vi "冰箱监测界面.vi"() -> ()   [LabVIEW 2016, in "环境动力监测库.lvlib"]
uses:
  <vilib>/ptbypt/NI_PtbyPt.lvlib
panel:
  out "关闭温度":dbl=40.0
  out "开启温度":dbl=50.0
  out "输出点":i32
  in  "控制开关":bool
  # "冰箱监测"
  # "℃"
  # "℃"
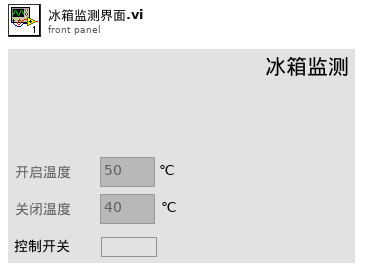
[diagram p1: front panel]
types:
  T1 = cluster{"环境变量":cluster{"蓄电池电压":dbl, "室温":dbl, "湿度":dbl, "水浸报警":bool, "烟雾报警":bool, "门禁1状态":bool, "门禁2状态":bool}, "ZLAN 6842 MB session":refnum<class "MB_Master.lvclass">, "DI":bool[], "DO":bool[]}
  T2 = cluster{"漏水监测配置":cluster{"监测项描述:输出":string, "端口":enum16{"AI0", "AI1", "AI2", "AI3", "AI4", "DI0", "DI1", "DI2", "DI3", "DI4", "DI5", "DI6", "DI7", "DO0", "DO1", "DO2", "DO3", "DO4", "DO5", "DO6", "DO7", "X0", "X1", "X2", "X3", "X4", "X5", "X6", "X7", "X8", "X9", "X10", "X11", "X12", "X13", "X14", "X15", "X16", "X17", "X18", "X19", "X20", "X21", "X22", "X23", "Y0", "Y1", "Y2", "Y3", "Y4", "Y5", "Y6", "Y7", "Y8", "Y9", "Y10", "Y11", "Y12", "Y13", "Y14", "Y15", "Y16", "Y17", "Y18", "Y19", "Y20", "Y21", "Y22", "Y23", "Y24", "Y25", "Y26", "Y27", "Y28", "Y29", "Y30", "Y31", "Y32", "Y33", "Y34", "Y35", "Y36", "Y37", "Y38", "Y39"}, "告警参数:":enum32{"禁用告警", "闭合告警", "断开告警"}, "传感器型号:":enum16{"PLC", "ZLAN", "ART"}, "声光告警启用":bool}, "门禁开关监测配置":cluster{"监测项描述:输出":string, "端口":enum16{"AI0", "AI1", "AI2", "AI3", "AI4", "DI0", "DI1", "DI2", "DI3", "DI4", "DI5", "DI6", "DI7", "DO0", "DO1", "DO2", "DO3", "DO4", "DO5", "DO6", "DO7", "X0", "X1", "X2", "X3", "X4", "X5", "X6", "X7", "X8", "X9", "X10", "X11", "X12", "X13", "X14", "X15", "X16", "X17", "X18", "X19", "X20", "X21", "X22", "X23", "Y0", "Y1", "Y2", "Y3", "Y4", "Y5", "Y6", "Y7", "Y8", "Y9", "Y10", "Y11", "Y12", "Y13", "Y14", "Y15", "Y16", "Y17", "Y18", "Y19", "Y20", "Y21", "Y22", "Y23", "Y24", "Y25", "Y26", "Y27", "Y28", "Y29", "Y30", "Y31", "Y32", "Y33", "Y34", "Y35", "Y36", "Y37", "Y38", "Y39"}, "告警参数:":enum32{"禁用告警", "闭合告警", "断开告警"}, "传感器型号:":enum16{"PLC", "ZLAN", "ART"}, "声光告警启用":bool}, "门禁开关监测配置2":cluster{"监测项描述:输出":string, "端口":enum16{"AI0", "AI1", "AI2", "AI3", "AI4", "DI0", "DI1", "DI2", "DI3", "DI4", "DI5", "DI6", "DI7", "DO0", "DO1", "DO2", "DO3", "DO4", "DO5", "DO6", "DO7", "X0", "X1", "X2", "X3", "X4", "X5", "X6", "X7", "X8", "X9", "X10", "X11", "X12", "X13", "X14", "X15", "X16", "X17", "X18", "X19", "X20", "X21", "X22", "X23", "Y0", "Y1", "Y2", "Y3", "Y4", "Y5", "Y6", "Y7", "Y8", "Y9", "Y10", "Y11", "Y12", "Y13", "Y14", "Y15", "Y16", "Y17", "Y18", "Y19", "Y20", "Y21", "Y22", "Y23", "Y24", "Y25", "Y26", "Y27", "Y28", "Y29", "Y30", "Y31", "Y32", "Y33", "Y34", "Y35", "Y36", "Y37", "Y38", "Y39"}, "告警参数:":enum32{"禁用告警", "闭合告警", "断开告警"}, "传感器型号:":enum16{"PLC", "ZLAN", "ART"}, "声光告警启用":bool}, "温湿度监测配置":cluster{"监测项描述:输出":string, "端口":enum16{"AI0", "AI1", "AI2", "AI3", "AI4", "DI0", "DI1", "DI2", "DI3", "DI4", "DI5", "DI6", "DI7", "DO0", "DO1", "DO2", "DO3", "DO4", "DO5", "DO6", "DO7", "X0", "X1", "X2", "X3", "X4", "X5", "X6", "X7", "X8", "X9", "X10", "X11", "X12", "X13", "X14", "X15", "X16", "X17", "X18", "X19", "X20", "X21", "X22", "X23", "Y0", "Y1", "Y2", "Y3", "Y4", "Y5", "Y6", "Y7", "Y8", "Y9", "Y10", "Y11", "Y12", "Y13", "Y14", "Y15", "Y16", "Y17", "Y18", "Y19", "Y20", "Y21", "Y22", "Y23", "Y24", "Y25", "Y26", "Y27", "Y28", "Y29", "Y30", "Y31", "Y32", "Y33", "Y34", "Y35", "Y36", "Y37", "Y38", "Y39"}, "告警参数:":enum32{"禁用告警", "闭合告警", "断开告警"}, "传感器型号:":enum16{"PLC", "ZLAN", "ART"}, "声光告警启用":bool}, "烟雾监测配置":cluster{"监测项描述:输出":string, "端口":enum16{"AI0", "AI1", "AI2", "AI3", "AI4", "DI0", "DI1", "DI2", "DI3", "DI4", "DI5", "DI6", "DI7", "DO0", "DO1", "DO2", "DO3", "DO4", "DO5", "DO6", "DO7", "X0", "X1", "X2", "X3", "X4", "X5", "X6", "X7", "X8", "X9", "X10", "X11", "X12", "X13", "X14", "X15", "X16", "X17", "X18", "X19", "X20", "X21", "X22", "X23", "Y0", "Y1", "Y2", "Y3", "Y4", "Y5", "Y6", "Y7", "Y8", "Y9", "Y10", "Y11", "Y12", "Y13", "Y14", "Y15", "Y16", "Y17", "Y18", "Y19", "Y20", "Y21", "Y22", "Y23", "Y24", "Y25", "Y26", "Y27", "Y28", "Y29", "Y30", "Y31", "Y32", "Y33", "Y34", "Y35", "Y36", "Y37", "Y38", "Y39"}, "告警参数:":enum32{"禁用告警", "闭合告警", "断开告警"}, "传感器型号:":enum16{"PLC", "ZLAN", "ART"}, "声光告警启用":bool}, "冰箱监测配置":cluster{"监测项描述:输出":string, "端口":enum16{"AI0", "AI1", "AI2", "AI3", "AI4", "DI0", "DI1", "DI2", "DI3", "DI4", "DI5", "DI6", "DI7", "DO0", "DO1", "DO2", "DO3", "DO4", "DO5", "DO6", "DO7", "X0", "X1", "X2", "X3", "X4", "X5", "X6", "X7", "X8", "X9", "X10", "X11", "X12", "X13", "X14", "X15", "X16", "X17", "X18", "X19", "X20", "X21", "X22", "X23", "Y0", "Y1", "Y2", "Y3", "Y4", "Y5", "Y6", "Y7", "Y8", "Y9", "Y10", "Y11", "Y12", "Y13", "Y14", "Y15", "Y16", "Y17", "Y18", "Y19", "Y20", "Y21", "Y22", "Y23", "Y24", "Y25", "Y26", "Y27", "Y28", "Y29", "Y30", "Y31", "Y32", "Y33", "Y34", "Y35", "Y36", "Y37", "Y38", "Y39"}, "告警参数:":enum32{"禁用告警", "闭合告警", "断开告警"}, "传感器型号:":enum16{"PLC", "ZLAN", "ART"}, "声光告警启用":bool}, "排气扇监测配置":cluster{"监测项描述:输出":string, "端口":enum16{"AI0", "AI1", "AI2", "AI3", "AI4", "DI0", "DI1", "DI2", "DI3", "DI4", "DI5", "DI6", "DI7", "DO0", "DO1", "DO2", "DO3", "DO4", "DO5", "DO6", "DO7", "X0", "X1", "X2", "X3", "X4", "X5", "X6", "X7", "X8", "X9", "X10", "X11", "X12", "X13", "X14", "X15", "X16", "X17", "X18", "X19", "X20", "X21", "X22", "X23", "Y0", "Y1", "Y2", "Y3", "Y4", "Y5", "Y6", "Y7", "Y8", "Y9", "Y10", "Y11", "Y12", "Y13", "Y14", "Y15", "Y16", "Y17", "Y18", "Y19", "Y20", "Y21", "Y22", "Y23", "Y24", "Y25", "Y26", "Y27", "Y28", "Y29", "Y30", "Y31", "Y32", "Y33", "Y34", "Y35", "Y36", "Y37", "Y38", "Y39"}, "告警参数:":enum32{"禁用告警", "闭合告警", "断开告警"}, "传感器型号:":enum16{"PLC", "ZLAN", "ART"}, "声光告警启用":bool}, "红外入侵监测配置":cluster{"监测项描述:输出":string, "端口":enum16{"AI0", "AI1", "AI2", "AI3", "AI4", "DI0", "DI1", "DI2", "DI3", "DI4", "DI5", "DI6", "DI7", "DO0", "DO1", "DO2", "DO3", "DO4", "DO5", "DO6", "DO7", "X0", "X1", "X2", "X3", "X4", "X5", "X6", "X7", "X8", "X9", "X10", "X11", "X12", "X13", "X14", "X15", "X16", "X17", "X18", "X19", "X20", "X21", "X22", "X23", "Y0", "Y1", "Y2", "Y3", "Y4", "Y5", "Y6", "Y7", "Y8", "Y9", "Y10", "Y11", "Y12", "Y13", "Y14", "Y15", "Y16", "Y17", "Y18", "Y19", "Y20", "Y21", "Y22", "Y23", "Y24", "Y25", "Y26", "Y27", "Y28", "Y29", "Y30", "Y31", "Y32", "Y33", "Y34", "Y35", "Y36", "Y37", "Y38", "Y39"}, "告警参数:":enum32{"禁用告警", "闭合告警", "断开告警"}, "传感器型号:":enum16{"PLC", "ZLAN", "ART"}, "声光告警启用":bool}, "振动监测配置":cluster{"监测项描述:输出":string, "端口":enum16{"AI0", "AI1", "AI2", "AI3", "AI4", "DI0", "DI1", "DI2", "DI3", "DI4", "DI5", "DI6", "DI7", "DO0", "DO1", "DO2", "DO3", "DO4", "DO5", "DO6", "DO7", "X0", "X1", "X2", "X3", "X4", "X5", "X6", "X7", "X8", "X9", "X10", "X11", "X12", "X13", "X14", "X15", "X16", "X17", "X18", "X19", "X20", "X21", "X22", "X23", "Y0", "Y1", "Y2", "Y3", "Y4", "Y5", "Y6", "Y7", "Y8", "Y9", "Y10", "Y11", "Y12", "Y13", "Y14", "Y15", "Y16", "Y17", "Y18", "Y19", "Y20", "Y21", "Y22", "Y23", "Y24", "Y25", "Y26", "Y27", "Y28", "Y29", "Y30", "Y31", "Y32", "Y33", "Y34", "Y35", "Y36", "Y37", "Y38", "Y39"}, "告警参数:":enum32{"禁用告警", "闭合告警", "断开告警"}, "传感器型号:":enum16{"PLC", "ZLAN", "ART"}, "声光告警启用":bool}, "废液监测配置":cluster{"监测项描述:输出":string, "端口":enum16{"AI0", "AI1", "AI2", "AI3", "AI4", "DI0", "DI1", "DI2", "DI3", "DI4", "DI5", "DI6", "DI7", "DO0", "DO1", "DO2", "DO3", "DO4", "DO5", "DO6", "DO7", "X0", "X1", "X2", "X3", "X4", "X5", "X6", "X7", "X8", "X9", "X10", "X11", "X12", "X13", "X14", "X15", "X16", "X17", "X18", "X19", "X20", "X21", "X22", "X23", "Y0", "Y1", "Y2", "Y3", "Y4", "Y5", "Y6", "Y7", "Y8", "Y9", "Y10", "Y11", "Y12", "Y13", "Y14", "Y15", "Y16", "Y17", "Y18", "Y19", "Y20", "Y21", "Y22", "Y23", "Y24", "Y25", "Y26", "Y27", "Y28", "Y29", "Y30", "Y31", "Y32", "Y33", "Y34", "Y35", "Y36", "Y37", "Y38", "Y39"}, "告警参数:":enum32{"禁用告警", "闭合告警", "断开告警"}, "传感器型号:":enum16{"PLC", "ZLAN", "ART"}, "声光告警启用":bool}, "废液监测配置2":cluster{"监测项描述:输出":string, "端口":enum16{"AI0", "AI1", "AI2", "AI3", "AI4", "DI0", "DI1", "DI2", "DI3", "DI4", "DI5", "DI6", "DI7", "DO0", "DO1", "DO2", "DO3", "DO4", "DO5", "DO6", "DO7", "X0", "X1", "X2", "X3", "X4", "X5", "X6", "X7", "X8", "X9", "X10", "X11", "X12", "X13", "X14", "X15", "X16", "X17", "X18", "X19", "X20", "X21", "X22", "X23", "Y0", "Y1", "Y2", "Y3", "Y4", "Y5", "Y6", "Y7", "Y8", "Y9", "Y10", "Y11", "Y12", "Y13", "Y14", "Y15", "Y16", "Y17", "Y18", "Y19", "Y20", "Y21", "Y22", "Y23", "Y24", "Y25", "Y26", "Y27", "Y28", "Y29", "Y30", "Y31", "Y32", "Y33", "Y34", "Y35", "Y36", "Y37", "Y38", "Y39"}, "告警参数:":enum32{"禁用告警", "闭合告警", "断开告警"}, "传感器型号:":enum16{"PLC", "ZLAN", "ART"}, "声光告警启用":bool}}
  T3 = cluster{"监测项描述:输出":string, "端口":enum16{"AI0", "AI1", "AI2", "AI3", "AI4", "DI0", "DI1", "DI2", "DI3", "DI4", "DI5", "DI6", "DI7", "DO0", "DO1", "DO2", "DO3", "DO4", "DO5", "DO6", "DO7", "X0", "X1", "X2", "X3", "X4", "X5", "X6", "X7", "X8", "X9", "X10", "X11", "X12", "X13", "X14", "X15", "X16", "X17", "X18", "X19", "X20", "X21", "X22", "X23", "Y0", "Y1", "Y2", "Y3", "Y4", "Y5", "Y6", "Y7", "Y8", "Y9", "Y10", "Y11", "Y12", "Y13", "Y14", "Y15", "Y16", "Y17", "Y18", "Y19", "Y20", "Y21", "Y22", "Y23", "Y24", "Y25", "Y26", "Y27", "Y28", "Y29", "Y30", "Y31", "Y32", "Y33", "Y34", "Y35", "Y36", "Y37", "Y38", "Y39"}, "告警参数:":enum32{"禁用告警", "闭合告警", "断开告警"}, "传感器型号:":enum16{"PLC", "ZLAN", "ART"}, "声光告警启用":bool}
  T4 = enum16{"AI0", "AI1", "AI2", "AI3", "AI4", "DI0", "DI1", "DI2", "DI3", "DI4", "DI5", "DI6", "DI7", "DO0", "DO1", "DO2", "DO3", "DO4", "DO5", "DO6", "DO7", "X0", "X1", "X2", "X3", "X4", "X5", "X6", "X7", "X8", "X9", "X10", "X11", "X12", "X13", "X14", "X15", "X16", "X17", "X18", "X19", "X20", "X21", "X22", "X23", "Y0", "Y1", "Y2", "Y3", "Y4", "Y5", "Y6", "Y7", "Y8", "Y9", "Y10", "Y11", "Y12", "Y13", "Y14", "Y15", "Y16", "Y17", "Y18", "Y19", "Y20", "Y21", "Y22", "Y23", "Y24", "Y25", "Y26", "Y27", "Y28", "Y29", "Y30", "Y31", "Y32", "Y33", "Y34", "Y35", "Y36", "Y37", "Y38", "Y39"}
  T5 = cluster{"温湿度":cluster{"状态":bool, "温度:":sgl, "湿度:":sgl, "详情  ":bool}, "空调":cluster{"状态":bool, "机柜温度:":sgl, "压缩机:":enum16{"停止", "运行"}, "电加热:":enum16{"停止", "运行"}, "详情  ":bool}, "排气扇":cluster{"排气扇":bool, "详情  ":bool}, "冰箱":cluster{"冰箱":bool, "详情  ":bool}}
  T6 = cluster{"状态":cluster{"R0":i16, "R1":i16, "R2":i16, "R3":i16, "R4":i16, "R5":i16, "R6":i16, "R7":i16, "R8":i16, "R9":i16, "R10":i16, "R11":i16, "R12":i16, "R13":i16, "R14":i16, "R15":i16, "R16":i16, "R17":i16, "R18":i16, "R19":i16, "R20":i16, "R21":i16, "R22":i16, "R23":i16, "R24":i16, "R25":i16, "R26":i16, "R27":i16, "R28":i16, "R29":i16, "R30":i16, "R31":i16, "R32":i16, "R33":i16, "R34":i16, "R35":i16, "R36":i16, "R37":i16, "R38":i16, "R39":i16}, "输入状态":bool[], "输出状态":bool[], "参数设置":cluster{"R100":i16, "R101":i16, "R102":i16, "R103":i16, "R104":i16, "R105":i16, "R106":i16, "R107":i16, "R108":i16, "R109":i16, "R110":i16, "R111":i16, "R112":i16, "R113":i16, "R114":i16, "R115":i16, "R116":i16, "R117":i16, "R118":i16, "R119":i16, "R120":i16, "R121":i16, "R122":i16, "R123":i16}, "转换值":cluster{"AD0":sgl, "AD1":sgl, "AD2":sgl, "AD3":sgl, "AD4":sgl, "AD5":sgl}}
  T7 = cluster{"状态":cluster{"R0":i16, "R1":i16, "R2":i16, "R3":i16, "R4":i16, "R5":i16, "R6":i16, "R7":i16, "R8":i16, "R9":i16, "R10":i16, "R11":i16, "R12":i16, "R13":i16, "R14":i16, "R15":i16, "R16":i16, "R17":i16, "R18":i16, "R19":i16, "R20":i16, "R21":i16, "R22":i16, "R23":i16, "R24":i16, "R25":i16, "R26":i16, "R27":i16, "R28":i16, "R29":i16, "R30":i16, "R31":i16, "R32":i16, "R33":i16, "R34":i16, "R35":i16, "R36":i16, "R37":i16, "R38":i16, "R39":i16, "R40":i16, "R41":i16, "R42":i16, "R43":i16, "R44":i16, "R45":i16, "R46":i16, "R47":i16, "R48":i16, "R49":i16, "R50":i16, "R51":i16, "R52":i16, "R53":i16, "R54":i16, "R55":i16, "R56":i16, "R57":i16, "R58":i16, "R59":i16, "R60":i16, "R61":i16, "R62":i16, "R63":i16, "R64":i16, "R65":i16, "R66":i16, "R67":i16, "R68":i16, "R69":i16}, "输入状态":bool[], "输出状态":bool[], "报警簇":bool[], "参数设置":cluster{"R100":i16, "R101":i16, "R102":i16, "R103":i16, "R104":i16, "R105":i16, "R106":i16, "R107":i16, "R108":i16, "R109":i16, "R110":i16, "R111":i16, "R112":i16, "R113":i16, "R114":i16, "R115":i16, "R116":i16, "R117":i16, "R118":i16, "R119":i16, "R120":i16, "R121":i16, "R122":i16, "R123":i16, "R124":i16}, "转换值":cluster{"AD0":sgl, "AD1":sgl, "AD2":sgl, "AD3":sgl, "AD4":sgl, "AD5":sgl}, "看门狗启用":bool, "氨氮模块名称":string, "总磷模块名称":string, "采配水模块类型":enum16{"V1", "V2", "V3", "V4", "室内V1", "室内V2"}}
  T8 = cluster{"AD0":dbl, "AD1":dbl, "AD2":dbl, "AD3":dbl, "AD4":dbl, "AD5":dbl, "AD6":dbl, "AD7":dbl}
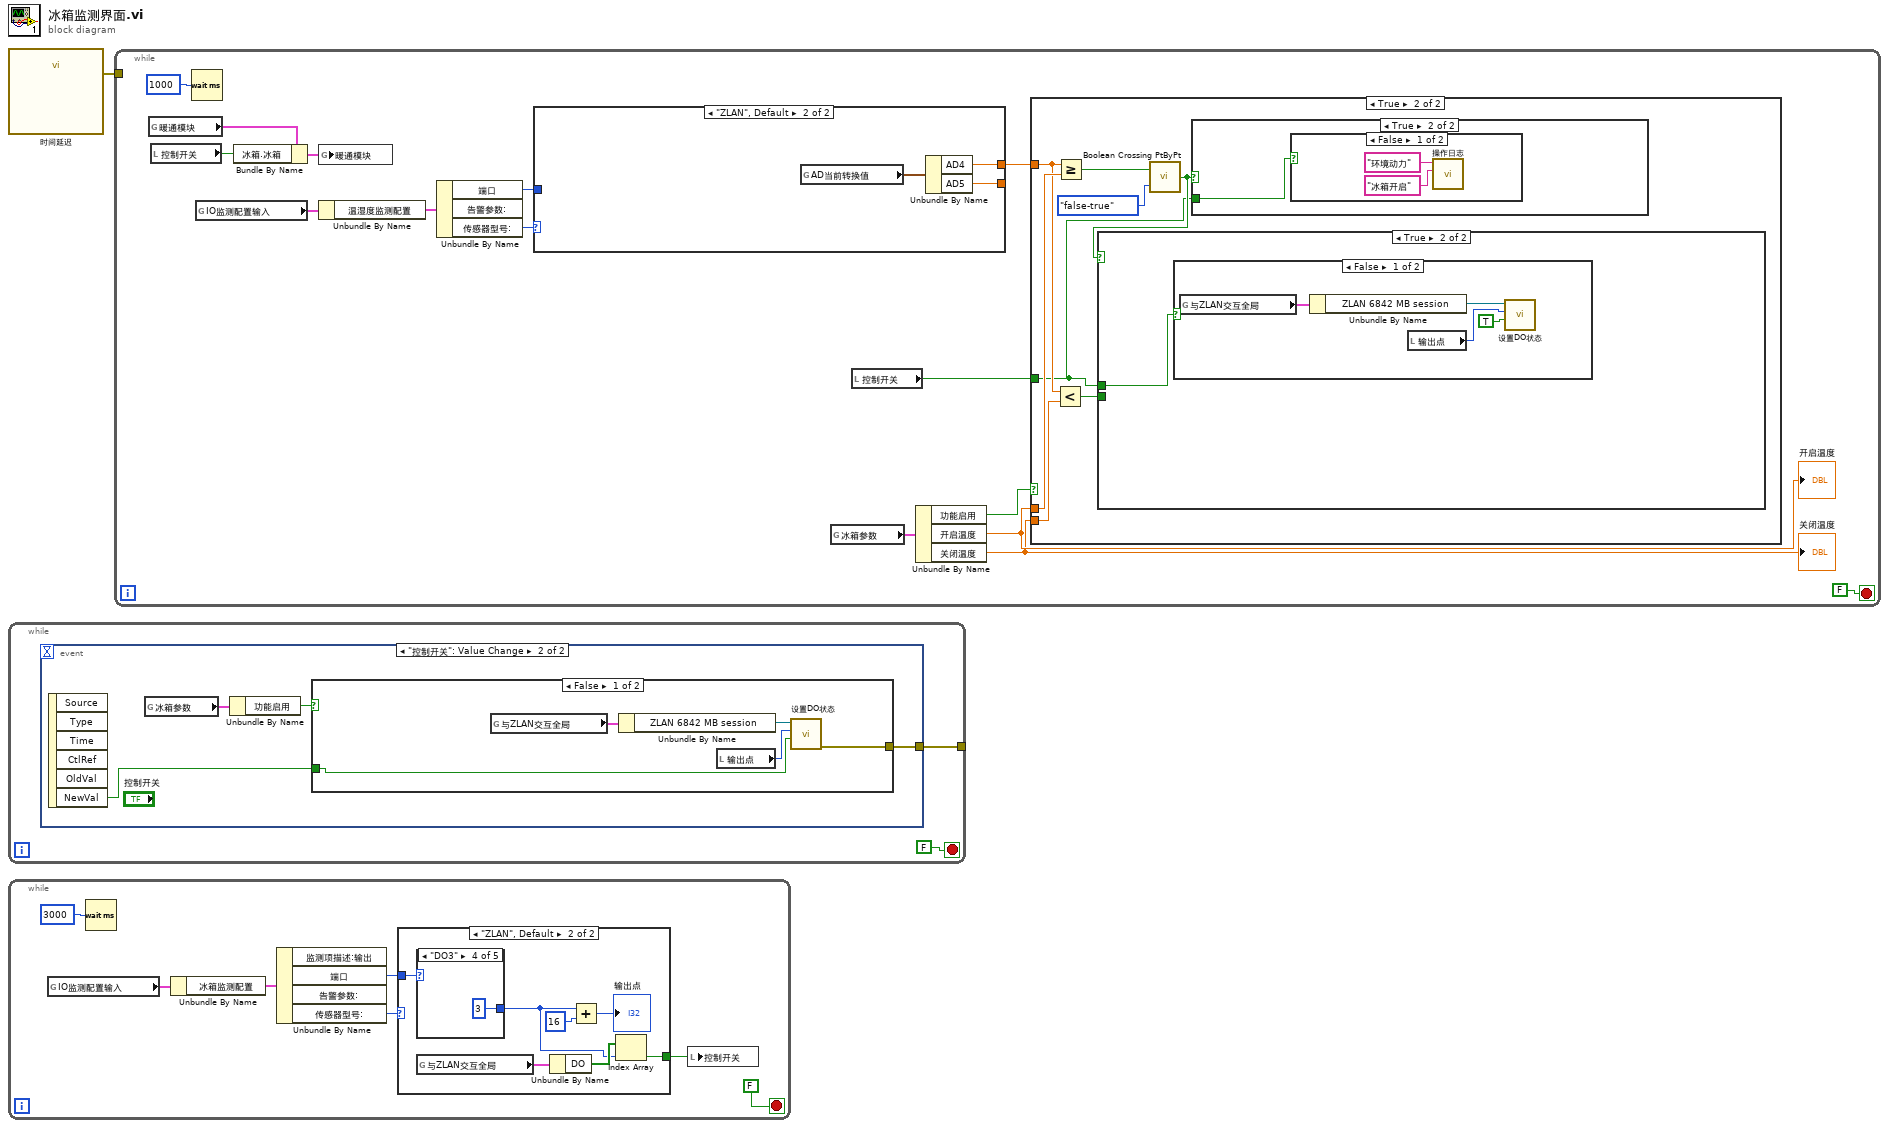
[diagram p0: block diagram]
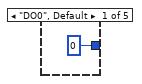
[diagram p3: hidden frame]
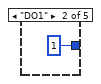
[diagram p4: hidden frame]
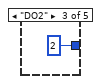
[diagram p5: hidden frame]
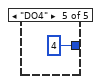
[diagram p6: hidden frame]
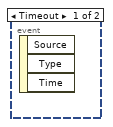
[diagram p7: hidden frame]
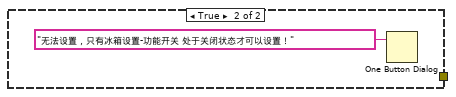
[diagram p8: hidden frame]
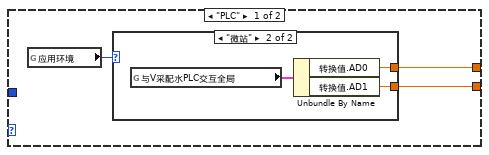
[diagram p9: hidden frame]
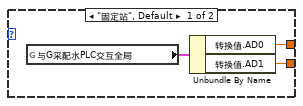
[diagram p10: hidden frame]
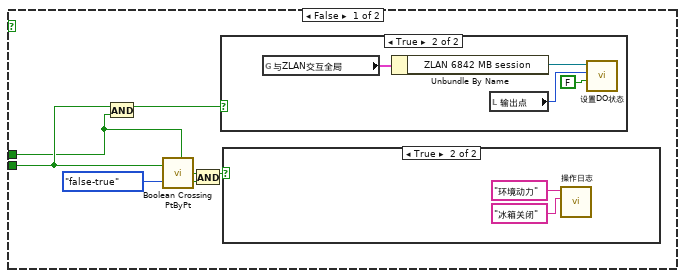
[diagram p12: hidden frame]
diagram:
  n1 = call "时间延迟"() -> ("error out"=w1:errorcluster)  [unwired: 11 in]
  n2 = while {
    tunnel: [w2] -> _
    stop <- FALSE stop-if-true
    n3 = event shown="[1] \"控制开关\": Value Change" {
      selector: _ -> [_ _]
      dyn-events: _ -> [_ _]
      timeout: _ -> [_ _]
      tunnel: [_ w4] -> w2
      event Timeout {
        n4 = event-data() -> ()  [unwired: 1 in, 3 out]
      }
      event "控制开关": Value Change {
        n5 = event-data() -> ("NewVal"=w5:bool)  [unwired: 1 in, 5 out]
        n6 = global read "断电保存全局变量.vi" "冰箱参数"() -> (w7:cluster{"功能启用":bool, "开启温度":dbl, "关闭温度":dbl})
        n7 = Unbundle By Name(w7) -> ("功能启用"=w6:bool)
        n8 = case shown="False" w6 {
          tunnel: w5 -> [w12 _]
          tunnel: [w11 _] -> w4
          frame False {
            n9 = global read "外部交互全局变量.vi" "与ZLAN交互全局"() -> (w10:T1)
            n10 = Unbundle By Name(w10) -> ("ZLAN 6842 MB session"=w9:refnum<class "MB_Master.lvclass">)
            n11 = local read "输出点"() -> (w8:i32)
            n12 = call "设置DO状态.vi"("value"=w12, "address"=w8, "MB session in"=w9) -> ("error out"=w11:errorcluster)  [unwired: 7 in, 1 out]
          }
          frame True {
            n13 = One Button Dialog(message="无法设置，只有冰箱设置-功能开关 处于关闭状态才可以设置！" ("消息")) -> ()  [unwired: 1 in, 1 out]
          }
        }
      }
    }
  }
  n14 = while {
    stop <- FALSE stop-if-true
    n15 = global read "断电保存全局变量.vi" "IO监测配置输入"() -> (w18:T2)
    n16 = Wait (ms)(milliseconds to wait=u32 3000 ("等待时间（毫秒）")) -> ()  [unwired: 1 out]
    n17 = Unbundle By Name(w18) -> ("冰箱监测配置"=w14:T3)
    n18 = Unbundle By Name(w14) -> ("端口"=w15:T4, "传感器型号:"=w16:enum16{"PLC", "ZLAN", "ART"})  [unwired: 2 out]
    n19 = case shown="\"ZLAN\", Default" w16 {
      tunnel: w15 -> [_ w27]
      tunnel: [_ w26] -> w17
      frame "PLC" {
      }
      frame "ZLAN", Default {
        n20 = case shown="\"DO3\"" w27 {
          tunnel: [0 1 2 3 4] -> w21
          frame "DO0", Default {
          }
          frame "DO1" {
          }
          frame "DO2" {
          }
          frame "DO3" {
          }
          frame "DO4" {
          }
        }
        n21 = global read "外部交互全局变量.vi" "与ZLAN交互全局"() -> (w25:T1)
        n22 = Unbundle By Name(w25) -> ("DO"=w24:bool[])
        n23 = Add(x=w21, y=16) -> (x+y=→"输出点":i32)
        n24 = Index Array(array=w24, index=w21) -> (element=w26:bool)
      }
    }
    n25 = local write "控制开关"(w17) -> ()
  }
  n26 = while {
    tunnel: w1 -> [_]
    stop <- FALSE stop-if-true
    n27 = global read "内部交互全局变量.vi" "暖通模块"() -> (w43:T5)
    n28 = local read "控制开关"() -> (w41:bool)
    n29 = Wait (ms)(milliseconds to wait=u32 1000 ("等待时间（毫秒）")) -> ()  [unwired: 1 out]
    n30 = global read "断电保存全局变量.vi" "IO监测配置输入"() -> (w36:T2)
    n31 = Bundle By Name(cluster=w43, "冰箱.冰箱"=w41) -> (w42:T5)
    n32 = global write "内部交互全局变量.vi" "暖通模块"(w42) -> ()
    n33 = Unbundle By Name(w36) -> ("温湿度监测配置"=w38:T3)
    n34 = Unbundle By Name(w38) -> ("端口"=w35:T4, "传感器型号:"=w37:enum16{"PLC", "ZLAN", "ART"})  [unwired: 1 out]
    n35 = case shown="\"ZLAN\", Default" w37 {
      tunnel: w35 -> [_ _]
      tunnel: [w49 w58] -> w34
      tunnel: [w48 w57] -> _
      frame "PLC" {
        n36 = global read "外部交互全局变量.vi" "应用环境"() -> (w50:enum16{"固定站", "微站", "浮标", "浮船"})
        n37 = case shown="\"微站\"" w50 {
          tunnel: [w52 w55] -> w49
          tunnel: [w51 w54] -> w48
          frame "固定站", Default {
            n38 = global read "外部交互全局变量.vi" "与G采配水PLC交互全局"() -> (w53:T6)
            n39 = Unbundle By Name(w53) -> ("转换值.AD0"=w52:sgl, "转换值.AD1"=w51:sgl)
          }
          frame "微站" {
            n40 = global read "外部交互全局变量.vi" "与V采配水PLC交互全局"() -> (w56:T7)
            n41 = Unbundle By Name(w56) -> ("转换值.AD0"=w55:sgl, "转换值.AD1"=w54:sgl)
          }
        }
      }
      frame "ZLAN", Default {
        n42 = global read "断电保存全局变量.vi" "AD当前转换值"() -> (w59:T8)
        n43 = Unbundle By Name(w59) -> ("AD4"=w58:dbl, "AD5"=w57:dbl)
      }
    }
    n44 = global read "断电保存全局变量.vi" "冰箱参数"() -> (w45:cluster{"功能启用":bool, "开启温度":dbl, "关闭温度":dbl})
    n45 = local read "控制开关"() -> (w33:bool)
    n46 = Unbundle By Name(w45) -> ("功能启用"=w44:bool, "开启温度"=w40:dbl, "关闭温度"=w39:dbl)
    "开启温度" <- w40
    "关闭温度" <- w39
    n47 = case shown="True" w44 {
      tunnel: w40 -> [_ w66]
      tunnel: w39 -> [_ w63]
      tunnel: w34 -> [_ w64]
      tunnel: w33 -> [_ w60]
      frame False {
      }
      frame True {
        n48 = Less?(x=w64, y=w63) -> (x < y?=w62:bool)
        n49 = Greater Or Equal?(x=w64, y=w66) -> (x >= y?=w65:bool)
        n50 = call <vilib>:"Boolean Crossing PtByPt.vi"("direction"=enum16{"either", "false-true", "true-false"}."false-true", "input"=w65) -> ("crossing"=w61:bool)  [unwired: 1 in]
        n51 = case shown="True" w61 {
          tunnel: w62 -> [w71 _]
          tunnel: w60 -> [w68 w80]
          frame False {
            n52 = And(x=w71, y=w68) -> (x .and. y?=w70:bool)
            n53 = call <vilib>:"Boolean Crossing PtByPt.vi"("direction"=enum16{"either", "false-true", "true-false"}."false-true", "input"=w71) -> ("crossing"=w72:bool)  [unwired: 1 in]
            n54 = And(x=w72, y=w68) -> (x .and. y?=w69:bool)
            n55 = case shown="True" w70 {
              frame False {
              }
              frame True {
                n56 = global read "外部交互全局变量.vi" "与ZLAN交互全局"() -> (w75:T1)
                n57 = Unbundle By Name(w75) -> ("ZLAN 6842 MB session"=w76:refnum<class "MB_Master.lvclass">)
                n58 = local read "输出点"() -> (w77:i32)
                n59 = call "设置DO状态.vi"("value"=FALSE, "address"=w77, "MB session in"=w76) -> ()  [unwired: 7 in, 2 out]
              }
            }
            n60 = case shown="True" w69 {
              frame False {
              }
              frame True {
                n61 = call "操作日志.vi"("日志信息"="冰箱关闭" ("设备"), "设备"="环境动力") -> ()  [unwired: 9 in, 1 out]
              }
            }
          }
          frame True {
            n62 = case shown="False" w80 {
              frame False {
                n63 = global read "外部交互全局变量.vi" "与ZLAN交互全局"() -> (w82:T1)
                n64 = Unbundle By Name(w82) -> ("ZLAN 6842 MB session"=w83:refnum<class "MB_Master.lvclass">)
                n65 = local read "输出点"() -> (w84:i32)
                n66 = call "设置DO状态.vi"("value"=TRUE, "address"=w84, "MB session in"=w83) -> ()  [unwired: 7 in, 2 out]
              }
              frame True {
              }
            }
          }
        }
        n67 = case shown="True" w61 {
          tunnel: w60 -> [_ w85]
          frame False {
          }
          frame True {
            n68 = case shown="False" w85 {
              frame False {
                n69 = call "操作日志.vi"("日志信息"="冰箱开启" ("设备"), "设备"="环境动力") -> ()  [unwired: 9 in, 1 out]
              }
              frame True {
              }
            }
          }
        }
      }
    }
  }
